vi "Write Relay State.vi"(8 "error in (no error)":errorcluster, 10 "Relay State":bool[](array[boolean]), 11 "SwitchMatrix in":refnum<class "SwitchMatrix.lvclass">) -> (0 "error out":errorcluster, 3 "SwitchMatrix out":refnum<class "SwitchMatrix.lvclass">)   [LabVIEW 2019, in "SwitchMatrix.lvlib" / "SwitchMatrix.lvclass"]
uses:
  Library/SwitchMatrix.lvclass
  Library/SwitchMatrix.lvclass/SwitchMatrix.ctl
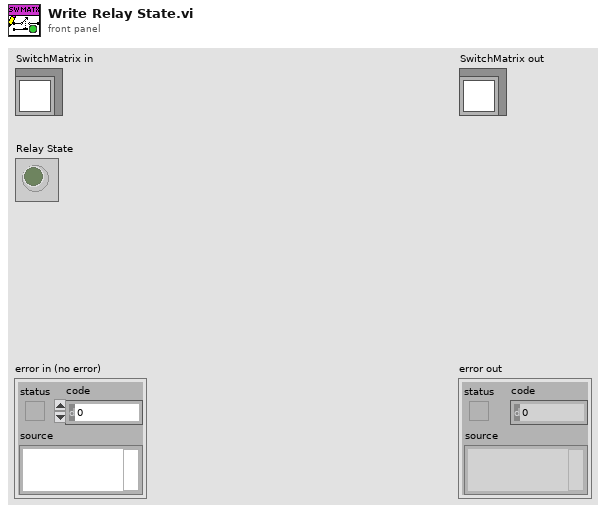
[diagram p1: front panel]
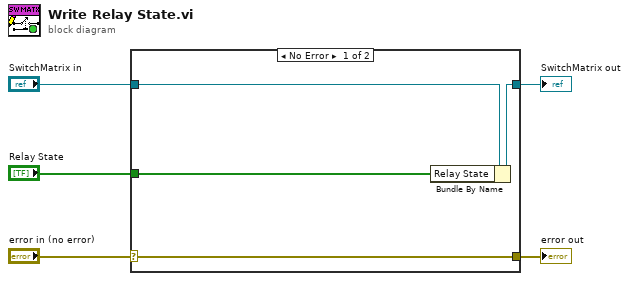
[diagram p0: block diagram]
diagram:
  n1 = case shown="No Error" "error in (no error)" {
    selector: "error in (no error)" -> [w9 w10]
    tunnel: [w9 w10] -> w4
    tunnel: [w7 w11] -> w2
    tunnel: "SwitchMatrix in" -> [w8 w11]
    tunnel: "Relay State" -> [w6 _]
    frame No Error {
      n2 = Bundle By Name(cluster=w8, "Relay State"=w6) -> (w7:refnum<class "SwitchMatrix.lvclass">)
    }
    frame Error {
    }
  }
  "error out" <- w4
  "SwitchMatrix out" <- w2
